vi "Get Connections Impl.vi"(4 "pin type":T1, 6 "site":i32, 8 "error in":errorcluster, 9 "session factory":refnum<class "ISession Factory.lvclass">, 10 "pin or relay names":string[](array[string]), 11 "session reservation in":refnum<class "Session Reservation.lvclass">) -> (0 "error out":errorcluster, 2 "connections":T2[](array[typedef]), 3 "session reservation out":refnum<class "Session Reservation.lvclass">)   [LabVIEW 2020, in "Measurement Plugin Session Management V1.lvlib" / "Session Reservation.lvclass"]
doc: "Validates if the <B> pin or relay names </B> reservation is successful and gets the connection information for the interested pins or pin groups."
uses:
  Session Reservation.lvclass
  Connection with Session.ctl
  Connection.ctl
  MeasurementLink Instrument/ISession Factory/ISession Factory.lvclass
  Pin Type.ctl
  Session Reservation.lvclass/Session Reservation.ctl
  MeasurementLink Measurement Server/Helpers/Error Strings Global Internal.vi
  <vilib>/Utility/error.llb/Error Cluster From Error Code.vi
  Connection Map/Connection Map.lvclass
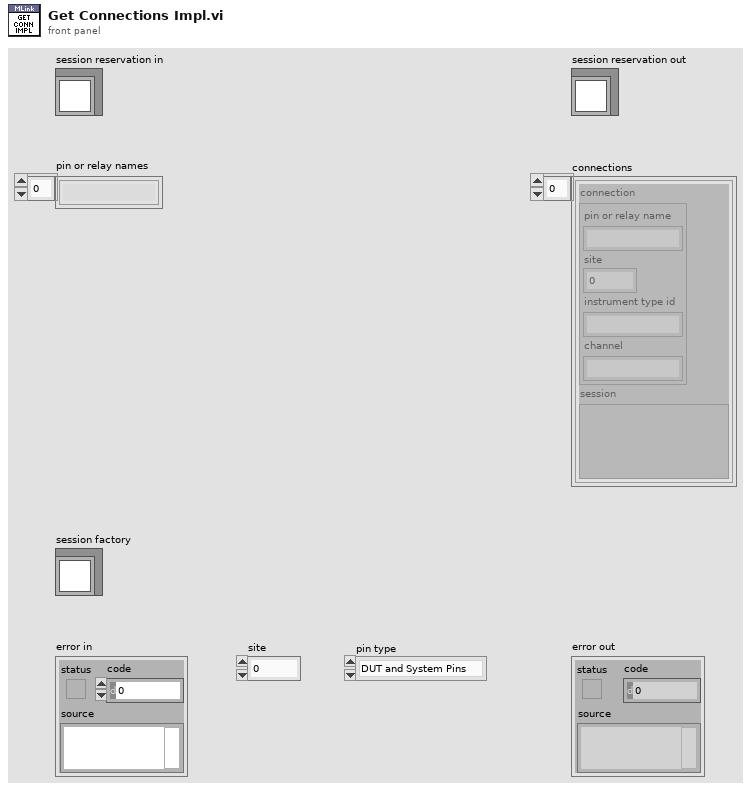
[diagram p1: front panel]
types:
  T1 = typedef "Measurement Plugin Session Management V1.lvlib/Session Reservation.lvclass/Pin Type.ctl" = enum16{"DUT and System Pins", "System Pins"}
  T2 = typedef "Measurement Plugin Session Management V1.lvlib/Session Reservation.lvclass/Connection with Session.ctl" = cluster{"connection":T3, "session":variant}
  T3 = typedef "Measurement Plugin Session Management V1.lvlib/Session Reservation.lvclass/Connection.ctl" = cluster{"pin or relay name":string, "site":i32, "instrument type id":string, "channel":string}
  T4 = typedef "Measurement Plugin Session Management V1.lvlib/Session Reservation.lvclass/Data.ctl" = cluster{"session and driver infos":T5[], "pin or relay names":string[], "connection map":refnum<class "Connection Map.lvclass">, "pin map context":T10, "reservation observer":refnum<class "IReservation Observer.lvclass">, "dvr valid":bool, "group mappings":T11}
  T5 = typedef "Measurement Plugin Session Management V1.lvlib/Session Reservation.lvclass/Session and Driver Info.ctl" = cluster{"session info":T6, "session":variant, "session factory":refnum<class "ISession Factory.lvclass">, "initialize and close session behavior":T9}
  T6 = typedef "MeasurementLink Session Management Client.lvlib/ni_measurementlink_sessionmanagement_v1_SessionInformation.ctl" = cluster{"session":T7, "resource_name":string, "channel_list":string, "instrument_type_id":string, "session_exists":bool, "channel_mappings":T8[]}
  T7 = typedef "MeasurementLink Session Management Client.lvlib/nidevice_grpc_Session.ctl" = cluster{"name":string}
  T8 = typedef "MeasurementLink Session Management Client.lvlib/ni_measurementlink_sessionmanagement_v1_ChannelMapping.ctl" = cluster{"pin_or_relay_name":string, "site":i32, "channel":string, "multiplexer_resource_name":string, "multiplexer_route":string}
  T9 = typedef "MeasurementLink Instrument.lvlib/ISession Factory.lvclass/Initialize and Close Session Behavior.ctl" = enum16{"Initialize and Close", "Attach and Detach", "Initialize and Detach", "Attach and Close"}
  T10 = typedef "MeasurementLink Session Management Client.lvlib/ni_measurementlink_PinMapContext.ctl" = cluster{"pin_map_id":string, "sites":i32[]}
  T11 = typedef "Measurement Plugin Session Management V1.lvlib/Session Reservation.lvclass/Group Mapping.ctl" = map{string, string[]}
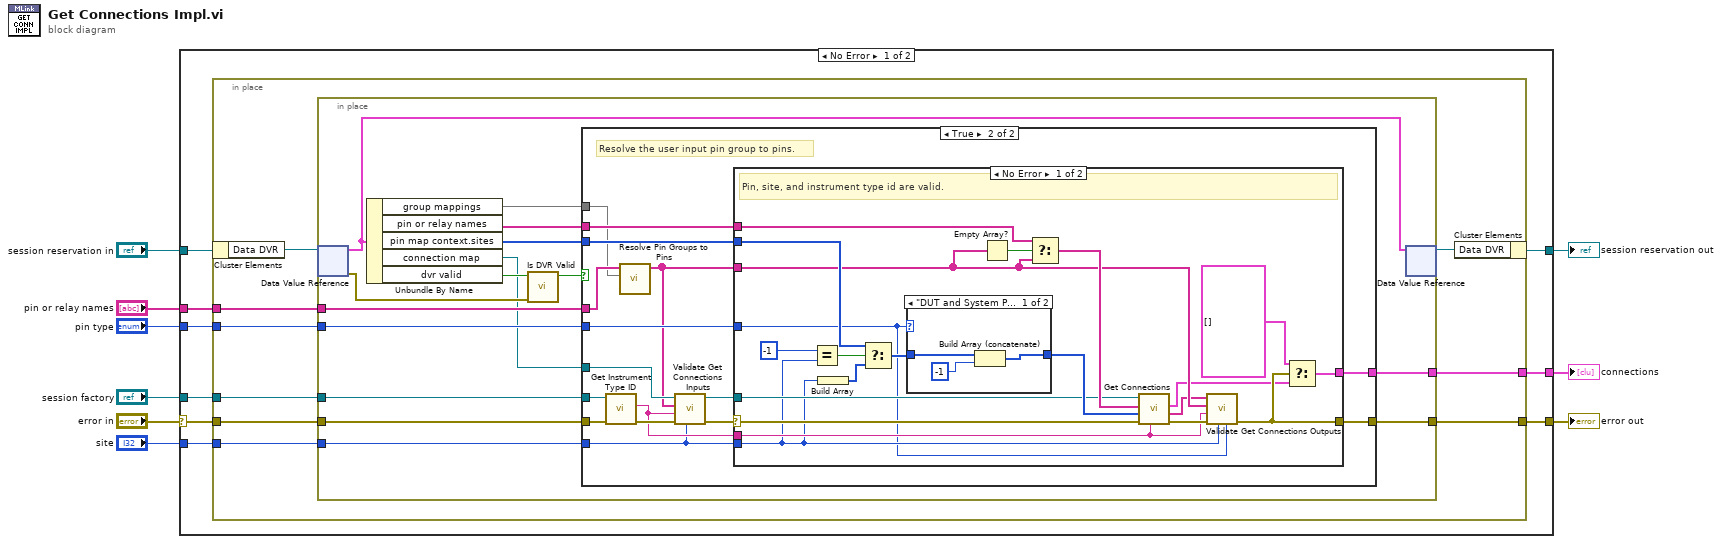
[diagram p0: block diagram]
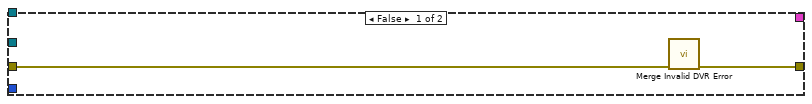
[diagram p2: hidden frame]
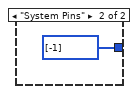
[diagram p3: hidden frame]
diagram:
  n1 = case shown="No Error" "error in" {
    selector: "error in" -> [w15 w88]
    tunnel: [w14 w88] -> w6
    tunnel: "session reservation in" -> [w12 w87]
    tunnel: "pin or relay names" -> [w18 _]
    tunnel: "site" -> [w17 _]
    tunnel: "session factory" -> [w16 _]
    tunnel: [w13 _] -> w4
    tunnel: [w11 w87] -> w2
    tunnel: "pin type" -> [w10 _]
    frame No Error {
      n2 = in-place {
        in-place-border: w18 -> [w27]
        in-place-border: w17 -> [w26]
        in-place-border: w16 -> [w25]
        in-place-border: w15 -> [w24]
        in-place-border: [w23] -> w14
        in-place-border: [w22] -> w13
        in-place-border: w10 -> [w19]
        n3 = in-place-cluster #1(w12) -> ("Data DVR"=w21:refnum<data-value>)
        n4 = in-place {
          in-place-border: w27 -> [w42]
          in-place-border: w26 -> [w41]
          in-place-border: w25 -> [w40]
          in-place-border: w24 -> [w39]
          in-place-border: [w38] -> w23
          in-place-border: [w37] -> w22
          in-place-border: w19 -> [w31]
          n5 = in-place-dvr #2(w21) -> (w32:T4, w34:errorcluster)
          n6 = Unbundle By Name(w32) -> ("group mappings"=w28:T11, "pin or relay names"=w36:string[], "pin map context.sites"=w35:i32[], "connection map"=w29:refnum<class "Connection Map.lvclass">, "dvr valid"=w30:bool)
          n7 = call "Is DVR Valid.vi"("dvr error in"=w34, "dvr valid in"=w30) -> ("dvr valid out"=w33:bool)  [unwired: 9 in]
          n8 = case shown="True" w33 {
            tunnel: w42 -> [_ w47]
            tunnel: w41 -> [_ w50]
            tunnel: w40 -> [_ w60]
            tunnel: w39 -> [w44 w59]
            tunnel: [w43 w58] -> w38
            tunnel: [_ w48] -> w37
            tunnel: w36 -> [_ w57]
            tunnel: w35 -> [_ w56]
            tunnel: w31 -> [_ w55]
            tunnel: w29 -> [_ w49]
            tunnel: w28 -> [_ w46]
            frame False {
              n9 = call "Merge Invalid DVR Error.vi"("error in"=w44) -> ("error out"=w43:errorcluster)  [unwired: 10 in]
            }
            frame True {
              # "Resolve the user input pin group to pins."
              n10 = call-dynamic "Get Instrument Type ID.vi"("error in"=w59, "session factory in"=w60) -> ("error out"=w54:errorcluster, "instrument type id"=w53:string)  [unwired: 7 in, 1 out]
              n11 = call "Resolve Pin Groups to Pins.vi"("group mappings"=w46, "pin or group names"=w47) -> ("resolved pin or relay names"=w45:string[])  [unwired: 9 in]
              n12 = call "Validate Get Connections Inputs.vi"("site"=w50, "error in"=w54, "instrument type id"=w53, "pin or relay names"=w45, "connection map"=w49) -> ("error out"=w52:errorcluster, "connection map out"=w51:refnum<class "Connection Map.lvclass">)  [unwired: 5 in]
              n13 = case shown="No Error" w52 {
                selector: w52 -> [w72 w86]
                tunnel: [w64 w86] -> w58
                tunnel: w57 -> [w77 _]
                tunnel: w56 -> [w75 _]
                tunnel: w55 -> [w65 _]
                tunnel: w53 -> [w67 _]
                tunnel: w51 -> [w71 _]
                tunnel: w45 -> [w69 _]
                tunnel: w50 -> [w66 _]
                tunnel: [w61 _] -> w48
                frame No Error {
                  # "Pin, site, and instrument type id are valid."
                  n14 = Equal?(x=-1, y=w66) -> (x = y?=w80:bool)
                  n15 = Build Array(w66) -> (w81:i32[])
                  n16 = Select(t=w75, s=w80, f=w81) -> (s? t:f=w74:i32[])
                  n17 = case shown="\"DUT and System Pins\"" w65 {
                    tunnel: w74 -> [w83 _]
                    tunnel: [w82 i32[] [-1] ("sites")] -> w73
                    frame "DUT and System Pins" {
                      n18 = Build Array (concatenate)(w83, -1 ("x")) -> (w82:i32[])
                    }
                    frame "System Pins" {
                    }
                  }
                  n19 = Empty Array?(array=w69) -> (empty?=w76:bool)
                  n20 = Select(t=w77, s=w76, f=w69) -> (s? t:f=w78:string[])
                  n21 = call "Get Connections.vi"("instrument type id"=w67, "error in"=w72, "sites"=w73, "pin or relay names"=w78, "connection map in"=w71) -> ("error out"=w70:errorcluster, "pin or relay names found"=w68:string[], "connections"=w63:T2[])  [unwired: 3 in, 1 out]
                  n22 = call "Validate Get Connections Outputs.vi"("pin type"=w65, "site"=w66, "error in"=w70, "instrument type id"=w67, "pin or relay names"=w69, "pin or relay names found"=w68) -> ("error out"=w64:errorcluster)  [unwired: 5 in]
                  n23 = Select(t=T2[] [], s=w64, f=w63) -> (s? t:f=w61:T2[])
                }
                frame Error {
                  # "Pin, site, or instrument type not in connections map."
                }
              }
            }
          }
          n24 = in-place-dvr #2(w32) -> (w20:refnum<data-value>)  [unwired: 1 out]
        }
        n25 = in-place-cluster #1("Data DVR"=w20) -> (w11:refnum<class "Session Reservation.lvclass">)
      }
    }
    frame Error {
    }
  }
  "error out" <- w6
  "connections" <- w4
  "session reservation out" <- w2
